vi "error - unknown section.vi"(8 "error in (no error)":errorcluster, 11 "section":string) -> (0 "error out":errorcluster)   [LabVIEW 2024, in "controls manager.lvlib"]
uses:
  controls manager.lvlib
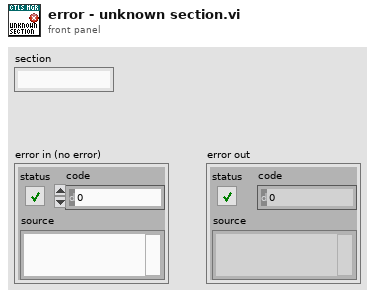
[diagram p1: front panel]
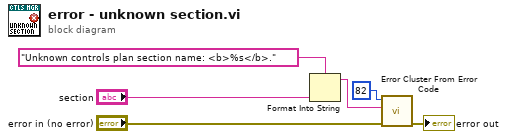
[diagram p0: block diagram]
diagram:
  n1 = Format Into String(format string="Unknown controls plan section name: <b>%s</b>.", "section") -> (resulting string=w2:string)  [unwired: 2 in, 1 out]
  n2 = call <vilib>:"Error Cluster From Error Code.vi"("error in (no error)"="error in (no error)", "error message (\"\")"=w2, "error code (0)"=82) -> ("error out"=→"error out":errorcluster)  [unwired: 6 in]
